vi "oa_Add Cursors on Cascade Plot.vi"(6 "grid color":u32(colorbox), 8 "order grids to display [order]":dbl[](array[numeric]), 10 "Y scale":cluster{"offset":dbl, "multiplier":dbl} {"multiplier" format="%.2f"; "offset" format="%.2f"}, 11 "waterfall plot":cluster{"X0":dbl, "dX":dbl, "Y":dbl[]}[](array[cluster]) {"Y" format="%.2f"; "dX" format="%.2f"; "X0" format="%.2f"}) -> (2 "cursor list":T1(array[cluster]), 3 "waterfall plot out":cluster{"X0":dbl, "dX":dbl, "Y":dbl[]}[](array[cluster]) {"Y" format="%.2f"; "dX" format="%.2f"; "X0" format="%.2f"})   [LabVIEW 2017]
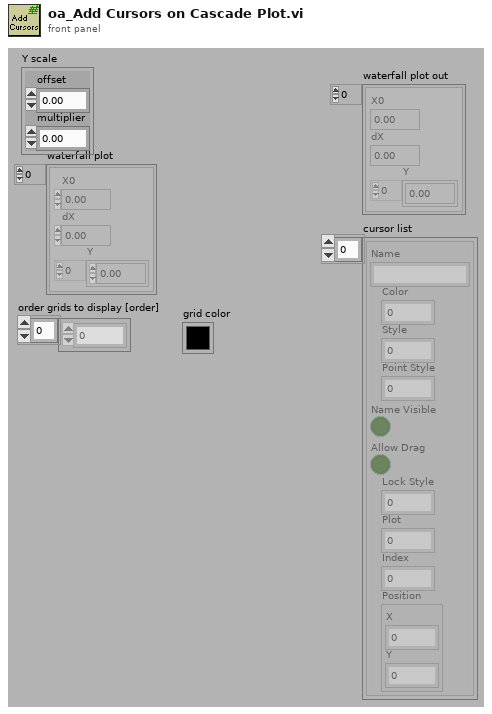
[diagram p1: front panel]
types:
  T1 = cluster{"Name":string, "Color":u32, "Style":u8, "Point Style":i32, "Name Visible":bool, "Allow Drag":bool, "Lock Style":i32, "Plot":u32, "Index":i32, "Position":cluster{"X":dbl, "Y":dbl}}[]
  T2 = cluster{"Name":string, "Color":u32, "Style":u8, "Point Style":i32, "Name Visible":bool, "Allow Drag":bool, "Lock Style":i32, "Plot":u32, "Index":i32, "Position":cluster{"X":dbl, "Y":dbl}}
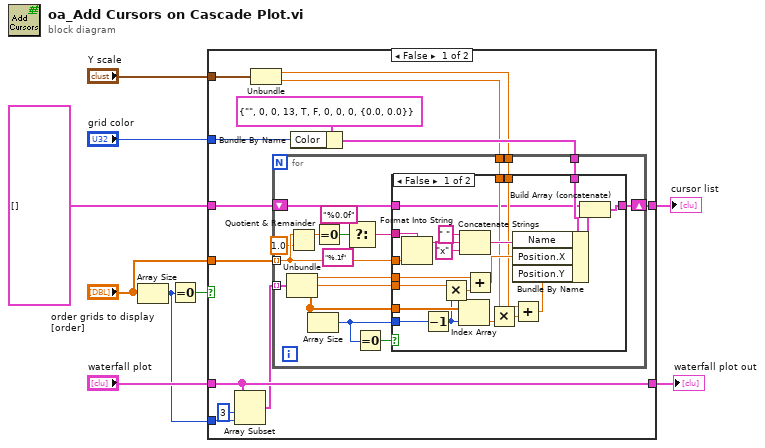
[diagram p0: block diagram]
diagram:
  n1 = Array Size(array="order grids to display [order]") -> (size(s)=w4:i32)
  n2 = Equal To 0?(x=w4) -> (x = 0?=w8:bool)
  n3 = case shown="False" w8 {
    tunnel: "grid color" -> [w21 _]
    tunnel: "order grids to display [order]" -> [w15 _]
    tunnel: "waterfall plot" -> [w19 w65]
    tunnel: [w19 w65] -> w6
    tunnel: w4 -> [w16 _]
    tunnel: "Y scale" -> [w14 _]
    tunnel: [w11 w64] -> w2
    tunnel: T1 [] -> [w10 w64]
    frame False {
      n4 = Array Subset(array=w19, index=3, length=w16) -> (w18:cluster{"X0":dbl, "dX":dbl, "Y":dbl[]}[])
      n5 = Unbundle(w14) -> ("offset"=w13:dbl, "multiplier"=w12:dbl)
      n6 = Bundle By Name(cluster=T2 {"Name"="", "Color"=0, "Style"=0, "Point Style"=13, "Name Visible"=TRUE, "Allow Drag"=FALSE, "Lock Style"=0, "Plot"=0, "Index"=0, "Position"={"X"=0.0, "Y"=0.0}}, "Color"=w21) -> (w17:T2)
      n7 = for {
        tunnel: w18 -> [w39] mode=indexing
        tunnel: w17 -> [w40]
        tunnel: w15 -> [w29] mode=indexing
        tunnel: w12 -> [w35]
        tunnel: w13 -> [w34]
        shift-right: [w31] -> w11
        shift-left: w10 -> [w30]
        n8 = Unbundle(w39) -> ("X0"=w37:dbl, "dX"=w36:dbl, "Y"=w38:dbl[])
        n9 = Quotient & Remainder(x=w29, y=1.0) -> (x-y*floor(x/y)=w27:dbl)  [unwired: 1 out]
        n10 = Array Size(array=w38) -> (size(s)=w33:i32)
        n11 = Equal To 0?(x=w27) -> (x = 0?=w26:bool)
        n12 = Select(t="%0.0f" ("format string"), s=w26, f="%.1f" ("format string")) -> (s? t:f=w23:string)
        n13 = Equal To 0?(x=w33) -> (x = 0?=w32:bool)
        n14 = case shown="False" w32 {
          tunnel: w40 -> [w62 _]
          tunnel: w29 -> [w58 _]
          tunnel: w38 -> [w56 _]
          tunnel: w37 -> [w55 _]
          tunnel: w36 -> [w54 _]
          tunnel: w33 -> [w53 _]
          tunnel: w35 -> [w50 _]
          tunnel: w34 -> [w47 _]
          tunnel: [w43 w63] -> w31
          tunnel: w30 -> [w42 w63]
          tunnel: w23 -> [w41 _]
          frame False {
            n15 = Format Into String(format string=w41, w58) -> (resulting string=w59:string)  [unwired: 2 in, 1 out]
            n16 = Decrement(x=w53) -> (x-1=w46:i32)
            n17 = Multiply(x=w54, y=w46) -> (x*y=w52:dbl)
            n18 = Index Array(array=w56, index=w46) -> (element=w49:dbl)
            n19 = Concatenate Strings(" " ("string"), w59, "x" ("string")) -> (w57:string)
            n20 = Add(x=w55, y=w52) -> (x+y=w51:dbl)
            n21 = Multiply(x=w50, y=w49) -> (x*y=w48:dbl)
            n22 = Add(x=w47, y=w48) -> (x+y=w45:dbl)
            n23 = Bundle By Name(cluster=w62, "Name"=w57, "Position.X"=w51, "Position.Y"=w45) -> (w44:T2)
            n24 = Build Array (concatenate)(w42, w44) -> (w43:T1)
          }
          frame True {
          }
        }
      }
    }
    frame True {
    }
  }
  "waterfall plot out" <- w6
  "cursor list" <- w2
